vi "FGV_REWORK_records_display.vi"(7 "options":T1, 8 "error_in":errorcluster, 11 "input":variant) -> (0 "error_out":errorcluster, 3 "output":variant)   [LabVIEW 2019]
uses:
  FGV_REWORK_records_display.ctl
  REWORK_references.ctl
  REWORK_all_info.ctl
  MAIN/REWORK_header_data_display.ctl
  REWORK_gear_statuses.ctl
  REWORK_gear_station.ctl
  _misc/AULocalize/SubVIs/Get Localized Phrase Compact Interface 0D.vi
  _misc/AULocalize/SubVIs/Get Localized Phrase Compact Interface 1D.vi
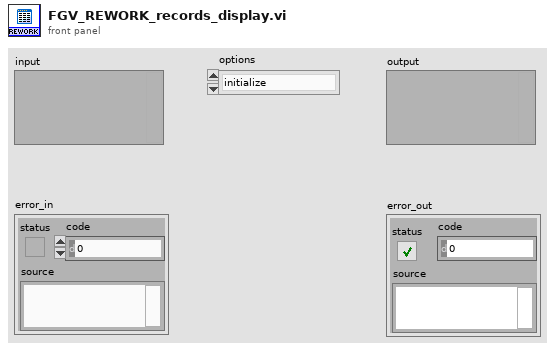
[diagram p1: front panel]
types:
  T1 = typedef "FGV_REWORK_records_display.ctl" = enum16{"initialize", "set_serial", "set_header", "set_operations", "set_results", "set_batches", "get_serial", "get_part_ID", "get_operation_IDs", "toggle_results", "show_all_results", "hide_all_results", "display", "clear"}
  T2 = typedef "REWORK_all_info.ctl" = cluster{"serial":string, "REWORK_header":T3, "operations":string[][], "operation_statuses":T4[], "results":string[][], "result_statuses":T4[], "batches":string[][], "batch_statuses":T4[], "REWORK_references":T5}
  T3 = typedef "REWORK_header_data_display.ctl" = cluster{"ID":string, "creation_time":string, "last_station":string, "last_status":string, "pinion_serial":string, "batch_code":string}
  T4 = typedef "REWORK_gear_statuses.ctl" = enum16{"OP_OK_hide", "OP_OK_show", "OP_NOK_hide", "OP_NOK_show", "OP_interrupted_hide", "OP_interrupted_show", "OP_in_operation_hide", "OP_in_operation_show", "OP_unexpected_hide", "OP_unexpected_show", "RE_REAL_OK", "RE_REAL_NOK", "RE_STRING", "RE_sub_header", "RE_no_data", "RE_unexpected", "BA_sub_header", "BA_data", "BA_no_data"}
  T5 = typedef "REWORK_references.ctl" = cluster{"front_panel_reference":refnum<vi>, "SQL_listbox_reference":refnum<vi>, "REWORK_header_data_display":refnum<vi>}
  T6 = typedef "REWORK_gear_station.ctl" = u16
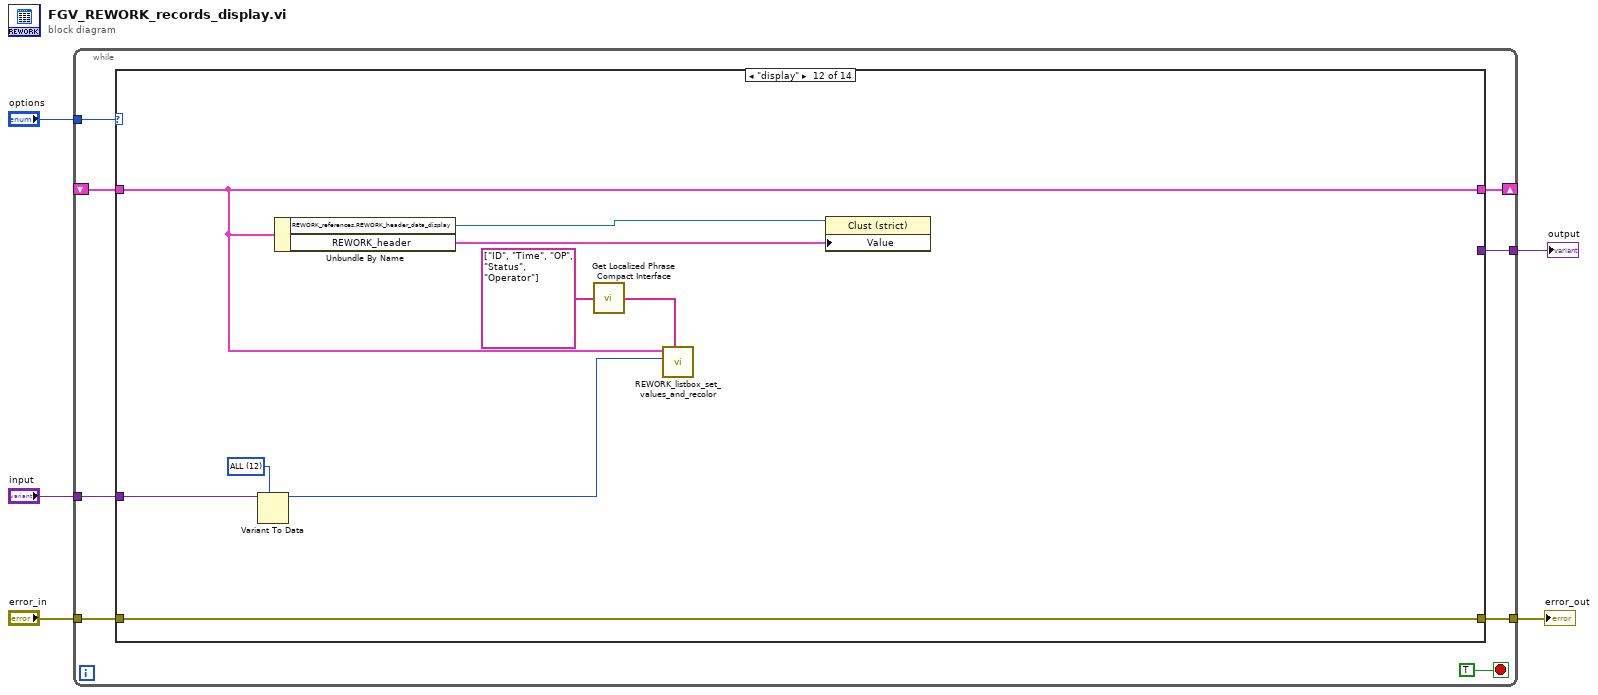
[diagram p0: block diagram]
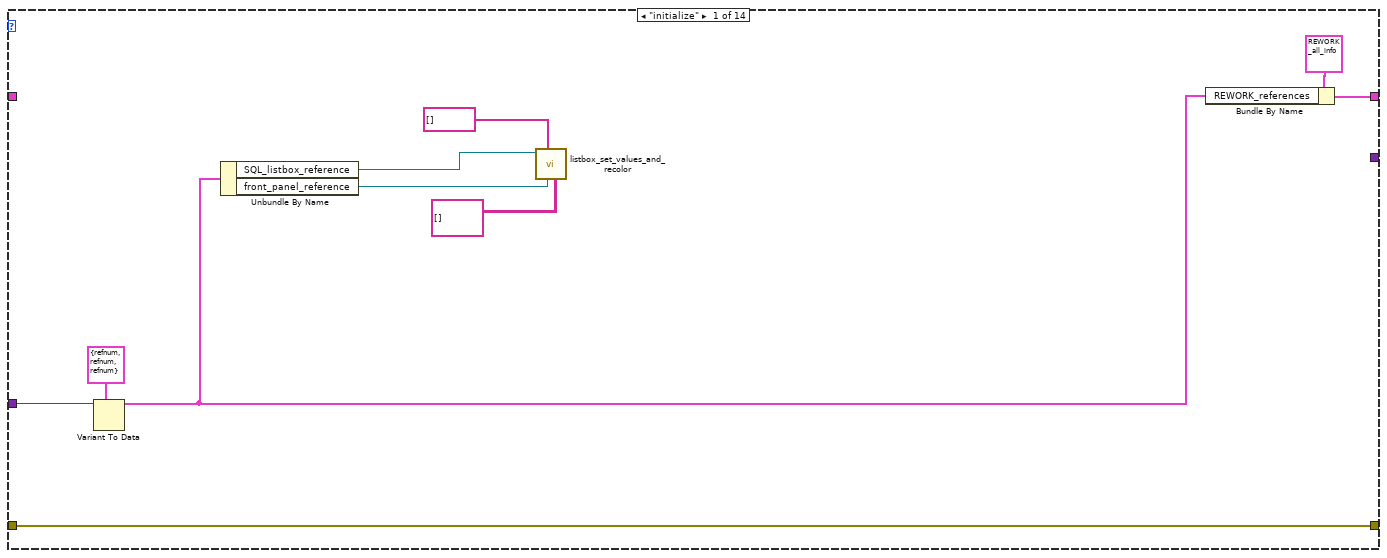
[diagram p2: hidden frame]
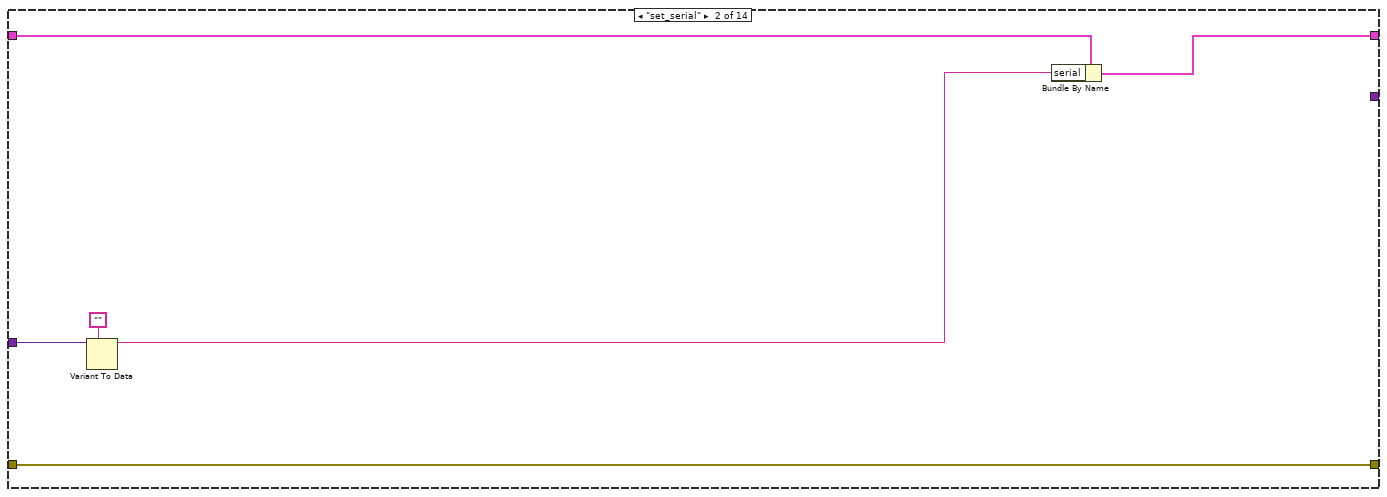
[diagram p3: hidden frame]
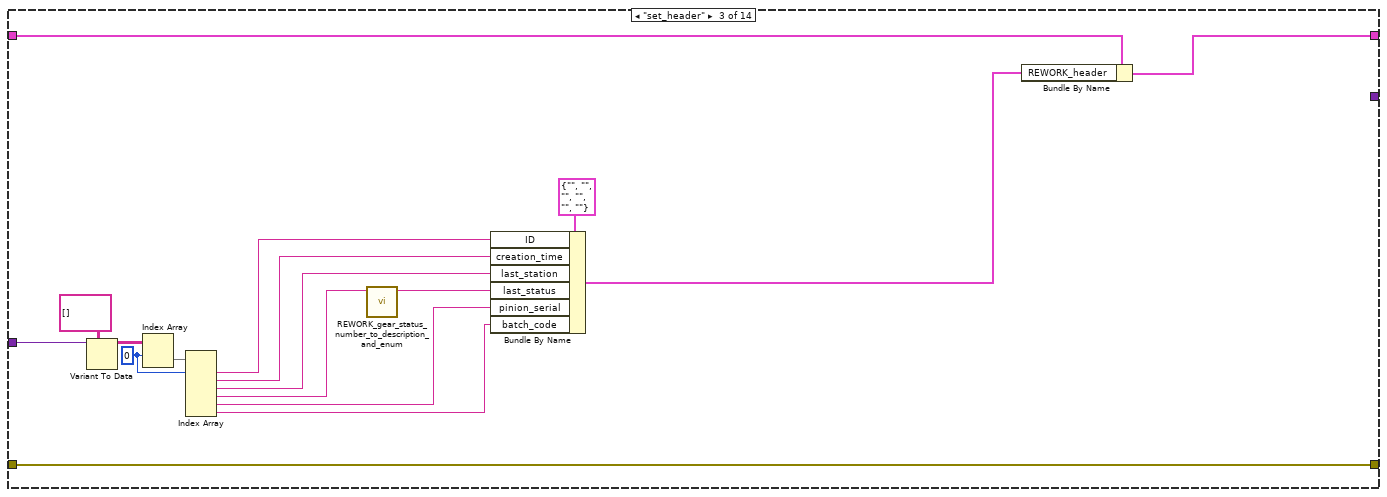
[diagram p4: hidden frame]
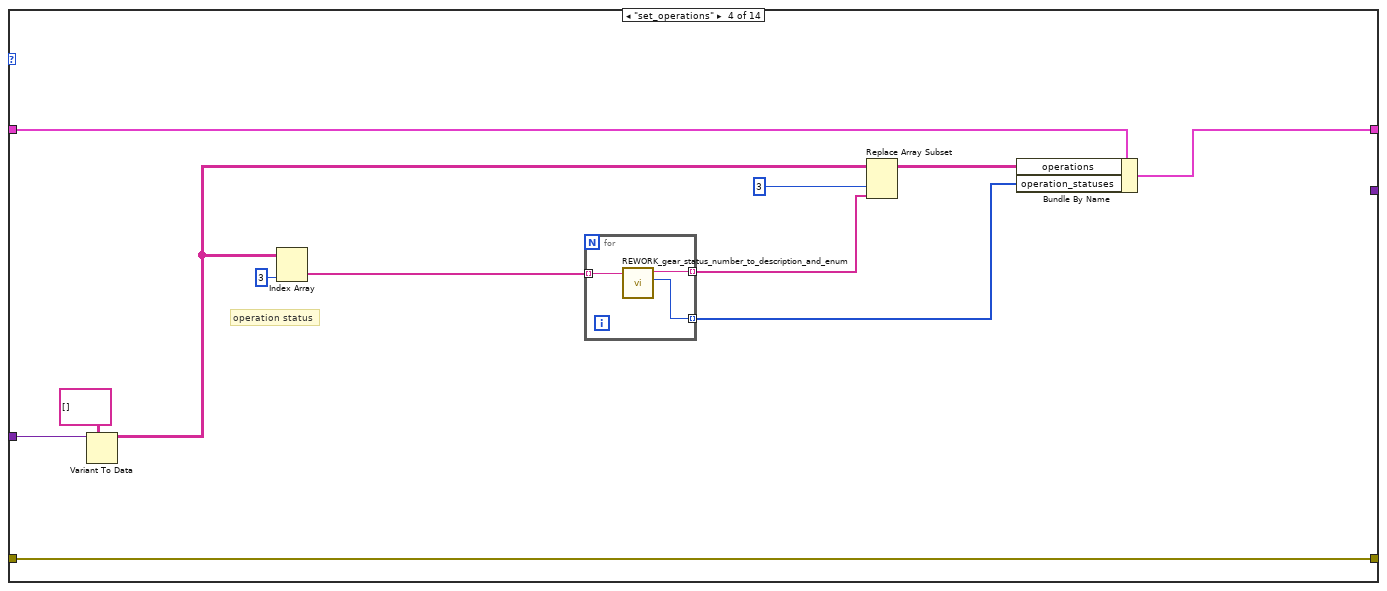
[diagram p5: hidden frame]
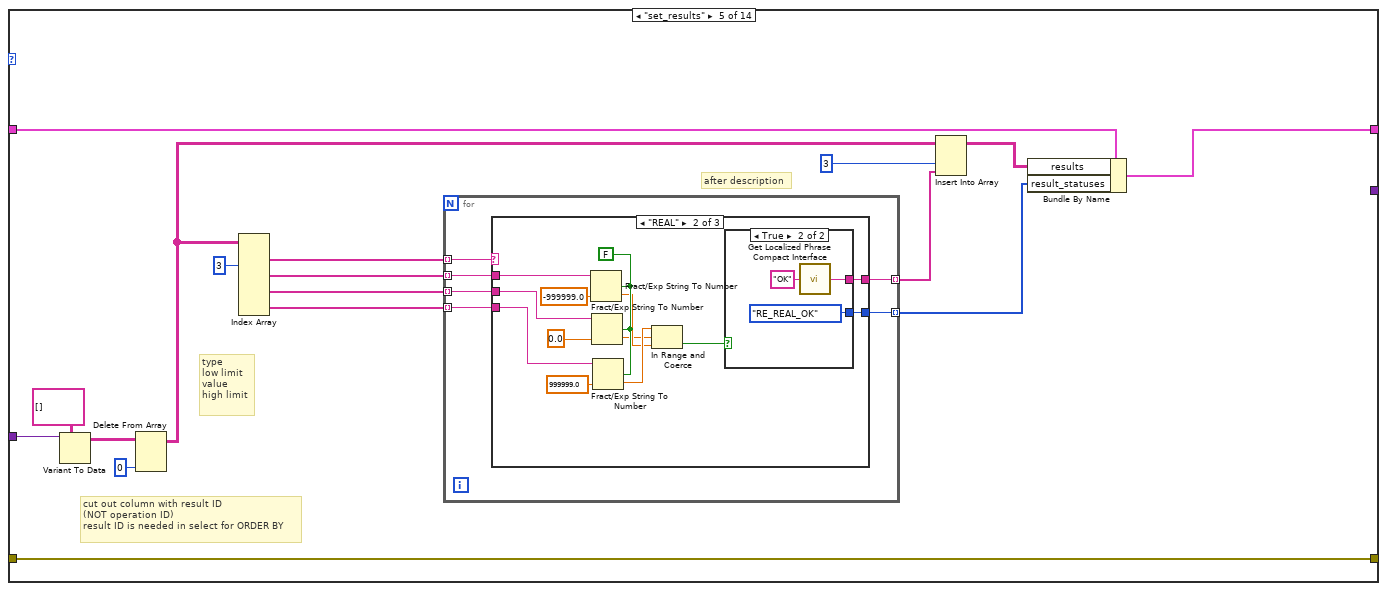
[diagram p6: hidden frame]
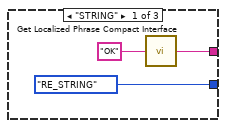
[diagram p7: hidden frame]
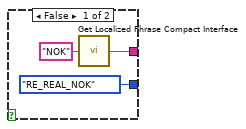
[diagram p8: hidden frame]
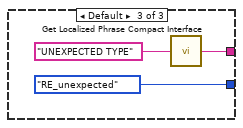
[diagram p9: hidden frame]
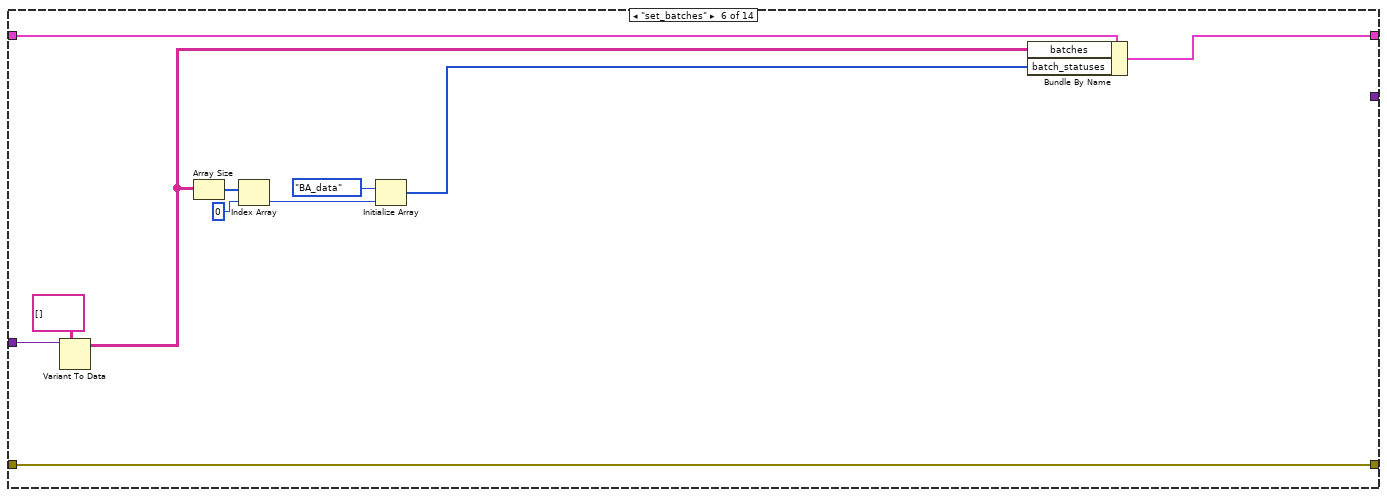
[diagram p10: hidden frame]
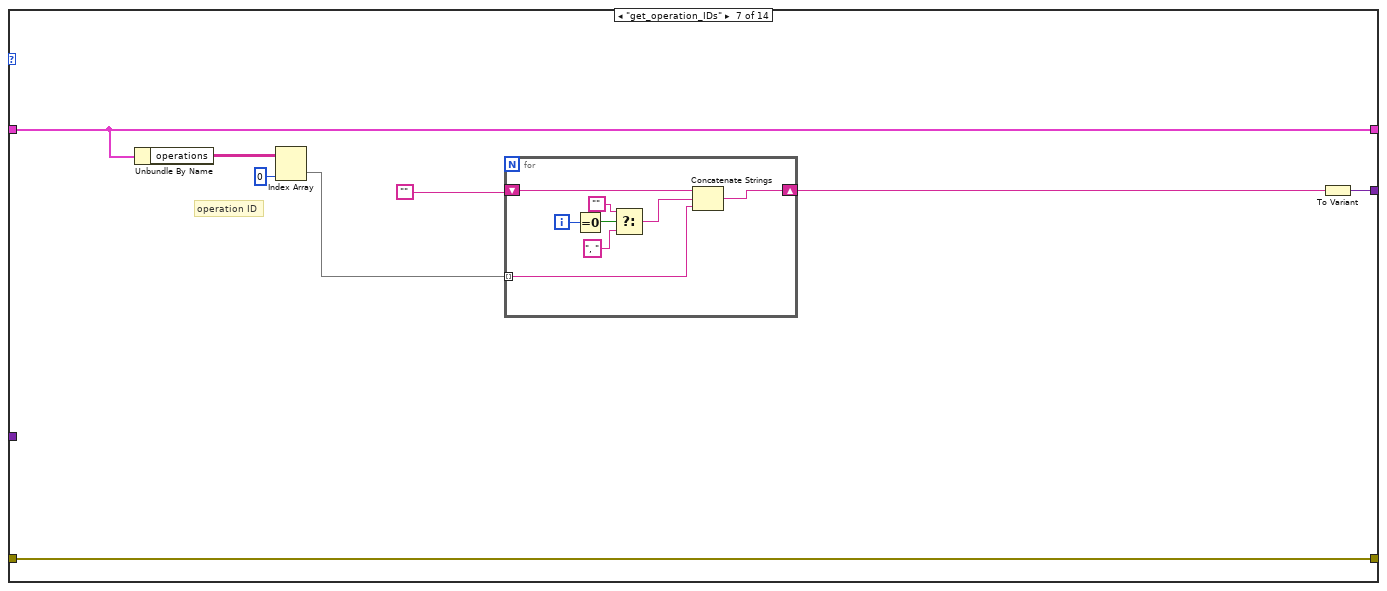
[diagram p11: hidden frame]
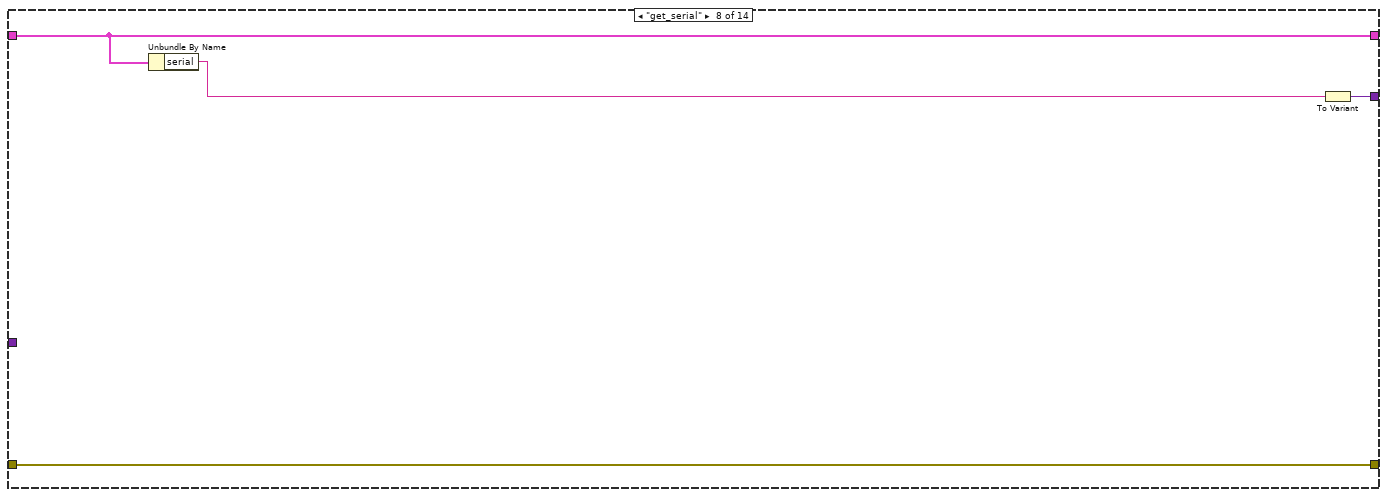
[diagram p12: hidden frame]
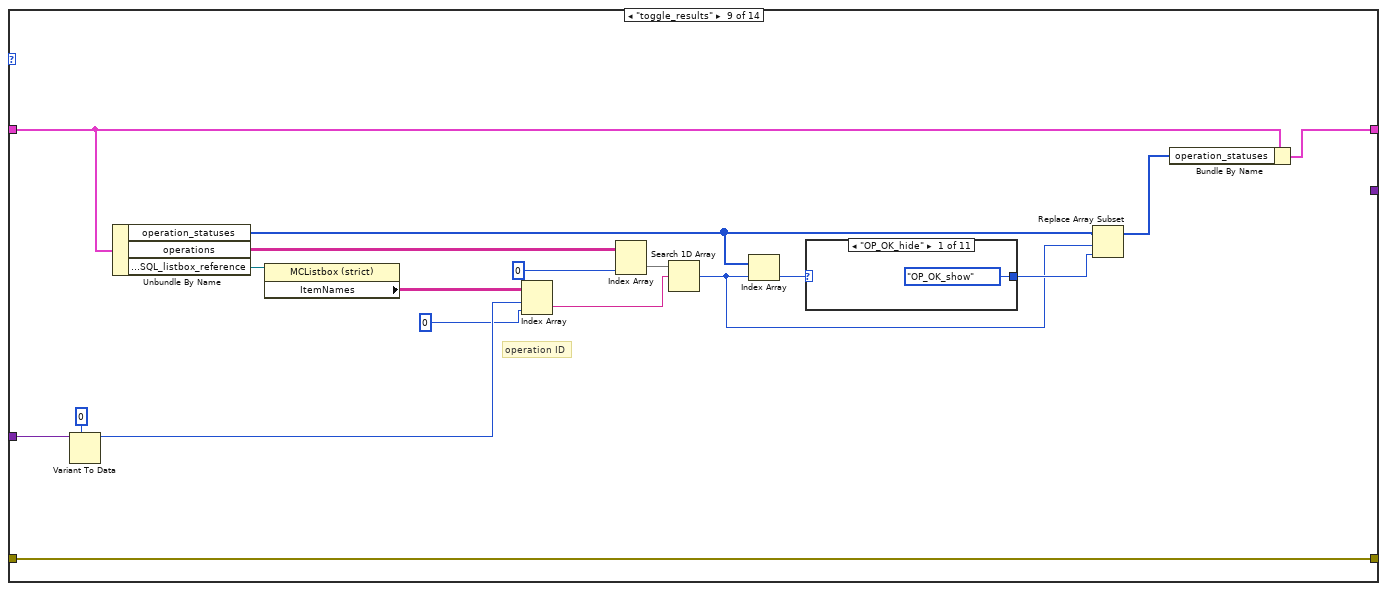
[diagram p13: hidden frame]
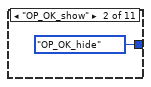
[diagram p14: hidden frame]
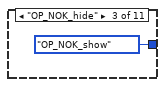
[diagram p15: hidden frame]
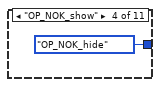
[diagram p16: hidden frame]
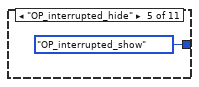
[diagram p17: hidden frame]
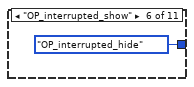
[diagram p18: hidden frame]
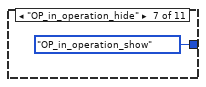
[diagram p19: hidden frame]
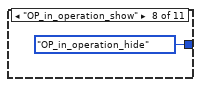
[diagram p20: hidden frame]
diagram:
  n1 = while {
    tunnel: "options" -> [w12]
    tunnel: [w11] -> w5
    tunnel: "error_in" -> [w10]
    shift-right: [w9] -> _
    shift-left: _ -> [w8]
    tunnel: "input" -> [w7]
    tunnel: [w6] -> w1
    stop <- TRUE stop-if-true
    n2 = case shown="\"display\"" w12 {
      tunnel: [w23 w29 w46 w58 w78 w120 w128 w140 w158 w174 w187 w204 w215 w216] -> w11
      tunnel: w10 -> [w23 w29 w46 w58 w78 w120 w128 w140 w158 w174 w187 w204 w215 w216]
      tunnel: [w15 w28 w45 w57 w77 w119 w126 w138 w142 w172 w185 w200 w208 w219] -> w9
      tunnel: w8 -> [_ w26 w43 w55 w75 w117 w126 w138 w143 w173 w186 w200 w212 w219]
      tunnel: w7 -> [w19 w27 w44 w56 w76 w118 _ _ w156 _ _ w199 _ _]
      tunnel: [_ _ _ _ _ _ w127 w139 _ _ _ _ _ w218] -> w6
      frame "initialize" {
        n3 = Variant To Data(type=T5 {"front_panel_reference"=refnum, "SQL_listbox_reference"=refnum, "REWORK_header_data_display"=refnum} ("REWORK_references"), Variant=w19) -> (data=w16:T5)  [unwired: 1 in, 1 out]
        n4 = Unbundle By Name(w16) -> ("SQL_listbox_reference"=w17:refnum<vi>, "front_panel_reference"=w18:refnum<vi>)
        n5 = call "listbox_set_values_and_recolor.vi"("item_names"=string[][] [], "front_panel_reference"=w18, "column_names"=string[] [], "multicolumn_listbox_reference_in"=w17) -> ()  [unwired: 6 in, 2 out]
        n6 = Bundle By Name(cluster=T2 {"serial"="", "REWORK_header"={"ID"="", "creation_time"="", "last_station"="", "last_status"="", "pinion_serial"="", "batch_code"=""}, "operations"=[], "operation_statuses"=[], "results"=[], "result_statuses"=[], "batches"=[], "batch_statuses"=[], "REWORK_references"={"front_panel_reference"=refnum, "SQL_listbox_reference"=refnum, "REWORK_header_data_display"=refnum}} ("REPORT_all_info"), "REWORK_references"=w16) -> (w15:T2)
      }
      frame "set_serial" {
        n7 = Variant To Data(type="", Variant=w27) -> (data=w24:string)  [unwired: 1 in, 1 out]
        n8 = Bundle By Name(cluster=w26, "serial"=w24) -> (w28:T2)
      }
      frame "set_header" {
        w38 = 0 ("index (row)")
        n9 = Variant To Data(type=string[][] [], Variant=w44) -> (data=w40:string[][])  [unwired: 1 in, 1 out]
        n10 = Index Array(array=w40, index (row)=w38) -> (element=w39:string[])  [unwired: 1 in]
        n11 = Index Array(array=w39, index #1=w38) -> (element #1=w36:string, element #2=w37:string, element #3=w35:string, element #4=w33:string, element #5=w34:string, element #6=w30:string)  [unwired: 5 in]
        n12 = call "REWORK_gear_status_number_to_description_and_enum.vi"("status_nmb"=w33) -> ("status_description"=w32:string)  [unwired: 9 in, 1 out]
        n13 = Bundle By Name(cluster=T3 {"ID"="", "creation_time"="", "last_station"="", "last_status"="", "pinion_serial"="", "batch_code"=""} ("REPORT_GEAR_header"), "ID"=w36, "creation_time"=w37, "last_station"=w35, "last_status"=w32, "pinion_serial"=w34, "batch_code"=w30) -> (w41:T3)
        n14 = Bundle By Name(cluster=w43, "REWORK_header"=w41) -> (w45:T2)
      }
      frame "set_operations" {
        # "operation status"
        n15 = Variant To Data(type=string[][] [], Variant=w56) -> (data=w50:string[][])  [unwired: 1 in, 1 out]
        n16 = Index Array(array=w50, index (col)=3 ("disabled index (col)")) -> (element=w52:string[])  [unwired: 1 in]
        n17 = for {
          tunnel: w52 -> [w61] mode=indexing
          tunnel: [w60] -> w51 mode=indexing
          tunnel: [w59] -> w47 mode=indexing
          n18 = call "REWORK_gear_status_number_to_description_and_enum.vi"("status_nmb"=w61) -> ("status_enum"=w60:T4, "status_description"=w59:string)  [unwired: 9 in]
        }
        n19 = Replace Array Subset(array=w50, new element=w47, index (col)=3 ("disabled index (col)")) -> (w48:string[][])  [unwired: 1 in]
        n20 = Bundle By Name(cluster=w55, "operations"=w48, "operation_statuses"=w51) -> (w57:T2)
      }
      frame "set_results" {
        # "after description"
        # "cut out column with result ID\n(NOT operation ID)\nresult ID is needed in select for ORDER BY"
        # "type\nlow limit\nvalue\nhigh limit"
        n21 = Variant To Data(type=string[][] [], Variant=w76) -> (data=w65:string[][])  [unwired: 1 in, 1 out]
        n22 = Delete From Array(array=w65, index (col)=0 ("disabled index (col)")) -> (array with subset deleted=w64:string[][])  [unwired: 2 in, 1 out]
        n23 = Index Array(array=w64, index (col) #1=3 ("disabled index (col)")) -> (element #1=w68:string[], element #2=w73:string[], element #3=w71:string[], element #4=w70:string[])  [unwired: 7 in]
        n24 = for {
          tunnel: w73 -> [w81] mode=indexing
          tunnel: [w84] -> w72 mode=indexing
          tunnel: [w83] -> w66 mode=indexing
          tunnel: w71 -> [w80] mode=indexing
          tunnel: w70 -> [w79] mode=indexing
          tunnel: w68 -> [w82] mode=indexing
          n25 = case shown="\"REAL\"" w82 {
            tunnel: [REWORK_gear_statuses."RE_STRING" ("REPORT_GEAR_statuses") w100 REWORK_gear_statuses."RE_unexpected" ("REPORT_GEAR_statuses")] -> w84
            tunnel: [w85 w99 w107] -> w83
            tunnel: w81 -> [_ w98 _]
            tunnel: w80 -> [_ w96 _]
            tunnel: w79 -> [_ w95 _]
            frame "STRING" {
              n26 = call-poly "Get Localized Phrase Compact Interface.vi"("Key"="OK") -> ("Translated Phrase"=w85:string)
            }
            frame "REAL" {
              w97 = FALSE ("use system decimal point (T)")
              n27 = Fract/Exp String To Number(use system decimal point (T)=w97, string=w98, default (0 dbl)=sgl -999999.0 ("default (0 DBL)")) -> (number=w93:sgl)  [unwired: 1 in, 1 out]
              n28 = Fract/Exp String To Number(use system decimal point (T)=w97, string=w96, default (0 dbl)=sgl 0.0 ("default (0 DBL)")) -> (number=w92:sgl)  [unwired: 1 in, 1 out]
              n29 = Fract/Exp String To Number(use system decimal point (T)=w97, string=w95, default (0 dbl)=sgl 999999.0 ("default (0 DBL)")) -> (number=w94:sgl)  [unwired: 1 in, 1 out]
              n30 = In Range and Coerce(upper limit=w94, x=w92, lower limit=w93) -> (In Range?=w91:bool)  [unwired: 1 out]
              n31 = case shown="True" w91 {
                tunnel: [REWORK_gear_statuses."RE_REAL_NOK" ("REPORT_GEAR_statuses") REWORK_gear_statuses."RE_REAL_OK" ("REPORT_GEAR_statuses")] -> w100
                tunnel: [w101 w104] -> w99
                frame False {
                  n32 = call-poly "Get Localized Phrase Compact Interface.vi"("Key"="NOK") -> ("Translated Phrase"=w101:string)
                }
                frame True {
                  n33 = call-poly "Get Localized Phrase Compact Interface.vi"("Key"="OK") -> ("Translated Phrase"=w104:string)
                }
              }
            }
            frame Default {
              n34 = call-poly "Get Localized Phrase Compact Interface.vi"("Key"="UNEXPECTED TYPE") -> ("Translated Phrase"=w107:string)
            }
          }
        }
        n35 = Insert Into Array(array=w64, index (col)=3 ("disabled index (col)"), new element=w66) -> (w67:string[][])  [unwired: 1 in]
        n36 = Bundle By Name(cluster=w75, "results"=w67, "result_statuses"=w72) -> (w77:T2)
      }
      frame "set_batches" {
        n37 = Variant To Data(type=string[][] [], Variant=w118) -> (data=w114:string[][])  [unwired: 1 in, 1 out]
        n38 = Array Size(array=w114) -> (size(s)=w113:i32[])
        n39 = Index Array(array=w113, index=0) -> (element=w111:i32)
        n40 = Initialize Array(REWORK_gear_statuses."BA_data" ("REPORT_GEAR_statuses"), w111) -> (w110:T4[])
        n41 = Bundle By Name(cluster=w117, "batches"=w114, "batch_statuses"=w110) -> (w119:T2)
      }
      frame "get_operation_IDs" {
        # "operation ID"
        n42 = Unbundle By Name(w126) -> ("operations"=w125:string[][])
        n43 = Index Array(array=w125, index (col)=0 ("disabled index (col)")) -> (element=w123:string[])  [unwired: 1 in]
        n44 = for {
          tunnel: w123 -> [w129] mode=indexing
          shift-right: [w132] -> w121
          shift-left: "" -> [w131]
          i -> [w133]
          n45 = Equal To 0?(x=w133) -> (x = 0?=w134:bool)
          n46 = Select(t="", s=w134, f=", ") -> (s? t:f=w130:string)
          n47 = Concatenate Strings(w131, w130, w129) -> (w132:string)
        }
        n48 = To Variant(anything=w121) -> (Variant=w127:variant)
      }
      frame "get_serial" {
        n49 = Unbundle By Name(w138) -> ("serial"=w137:string)
        n50 = To Variant(anything=w137) -> (Variant=w139:variant)
      }
      frame "toggle_results" {
        # "operation ID"
        n51 = Variant To Data(type=0 ("Row"), Variant=w156) -> (data=w153:i32)  [unwired: 1 in, 1 out]
        n52 = Unbundle By Name(w143) -> ("operation_statuses"=w146:T4[], "operations"=w151:string[][], "REWORK_references.SQL_listbox_reference"=w157:refnum<vi>)
        n53 = property class="MCListbox (strict)"(reference=w157) -> ("ItemNames"=w154:string[][])  [unwired: 1 in, 2 out]
        n54 = Index Array(array=w154, index (row)=w153, index (col)=0 ("disabled index (col)")) -> (element=w148:string)
        n55 = Index Array(array=w151, index (col)=0 ("disabled index (col)")) -> (element=w149:string[])  [unwired: 1 in]
        n56 = Search 1D Array(1D array=w149, element=w148) -> (index of element=w144:i32)  [unwired: 1 in]
        n57 = Index Array(array=w146, index=w144) -> (element=w147:T4)
        n58 = case shown="\"OP_OK_hide\"" w147 {
          selector: w147 -> [_ _ _ _ _ _ _ _ _ _ w169]
          tunnel: [REWORK_gear_statuses."OP_OK_show" ("REPORT_GEAR_statuses") REWORK_gear_statuses."OP_OK_hide" ("REPORT_GEAR_statuses") REWORK_gear_statuses."OP_NOK_show" ("REPORT_GEAR_statuses") REWORK_gear_statuses."OP_NOK_hide" ("REPORT_GEAR_statuses") REWORK_gear_statuses."OP_interrupted_show" ("REPORT_GEAR_statuses") REWORK_gear_statuses."OP_interrupted_hide" ("REPORT_GEAR_statuses") REWORK_gear_statuses."OP_in_operation_show" ("REPORT_GEAR_statuses") REWORK_gear_statuses."OP_in_operation_hide" ("REPORT_GEAR_statuses") REWORK_gear_statuses."OP_unexpected_show" ("REPORT_GEAR_statuses") REWORK_gear_statuses."OP_unexpected_hide" ("REPORT_GEAR_statuses") w169] -> w145
          frame "OP_OK_hide" {
          }
          frame "OP_OK_show" {
          }
          frame "OP_NOK_hide" {
          }
          frame "OP_NOK_show" {
          }
          frame "OP_interrupted_hide" {
          }
          frame "OP_interrupted_show" {
          }
          frame "OP_in_operation_hide" {
          }
          frame "OP_in_operation_show" {
          }
          frame "OP_unexpected_hide" {
          }
          frame "OP_unexpected_show" {
          }
          frame Default {
          }
        }
        n59 = Replace Array Subset(array=w146, new element=w145, index=w144) -> (w141:T4[])
        n60 = Bundle By Name(cluster=w143, "operation_statuses"=w141) -> (w142:T2)
      }
      frame "show_all_results" {
        n61 = Unbundle By Name(w173) -> ("operation_statuses"=w171:T4[])
        n62 = for {
          tunnel: w171 -> [w176] mode=indexing
          tunnel: [w175] -> w170 mode=indexing
          n63 = case shown="Default" w176 {
            selector: w176 -> [_ _ _ _ _ w182]
            tunnel: [REWORK_gear_statuses."OP_OK_show" ("REPORT_GEAR_statuses") REWORK_gear_statuses."OP_NOK_show" ("REPORT_GEAR_statuses") REWORK_gear_statuses."OP_interrupted_show" ("REPORT_GEAR_statuses") REWORK_gear_statuses."OP_in_operation_show" ("REPORT_GEAR_statuses") REWORK_gear_statuses."OP_unexpected_show" ("REPORT_GEAR_statuses") w182] -> w175
            frame "OP_OK_hide" {
            }
            frame "OP_NOK_hide" {
            }
            frame "OP_interrupted_hide" {
            }
            frame "OP_in_operation_hide" {
            }
            frame "OP_unexpected_hide" {
            }
            frame Default {
            }
          }
        }
        n64 = Bundle By Name(cluster=w173, "operation_statuses"=w170) -> (w172:T2)
      }
      frame "hide_all_results" {
        n65 = Unbundle By Name(w186) -> ("operation_statuses"=w184:T4[])
        n66 = for {
          tunnel: w184 -> [w188] mode=indexing
          tunnel: [w189] -> w183 mode=indexing
          n67 = case shown="\"OP_unexpected_show\"" w188 {
            selector: w188 -> [_ _ _ _ _ w195]
            tunnel: [REWORK_gear_statuses."OP_OK_hide" ("REPORT_GEAR_statuses") REWORK_gear_statuses."OP_NOK_hide" ("REPORT_GEAR_statuses") REWORK_gear_statuses."OP_interrupted_hide" ("REPORT_GEAR_statuses") REWORK_gear_statuses."OP_in_operation_hide" ("REPORT_GEAR_statuses") REWORK_gear_statuses."OP_unexpected_hide" ("REPORT_GEAR_statuses") w195] -> w189
            frame "OP_OK_show" {
            }
            frame "OP_NOK_show" {
            }
            frame "OP_interrupted_show" {
            }
            frame "OP_in_operation_show" {
            }
            frame "OP_unexpected_show" {
            }
            frame Default {
            }
          }
        }
        n68 = Bundle By Name(cluster=w186, "operation_statuses"=w183) -> (w185:T2)
      }
      frame "display" {
        w197 = T6 12 items=["Station 10", "Station 20", "Station 30", "Station 40", "Station 50", "Station 60", "Station 70", "Station 80", "Station 90", "Station 100", "Station 110", "Station 120", "ALL"] ("REPORT_GEAR_station")
        n69 = Variant To Data(type=w197, Variant=w199) -> (data=w198:T6)  [unwired: 1 in, 1 out]
        n70 = Unbundle By Name(w200) -> ("REWORK_references.REWORK_header_data_display"=w203:refnum<vi>, "REWORK_header"=w202:T3)
        n71 = call-poly "Get Localized Phrase Compact Interface.vi"("Key"=string[] ["ID", "Time", "OP", "Status", "Operator"] ("column_names")) -> ("Translated Phrase"=w196:string[])
        n72 = call "REWORK_listbox_set_values_and_recolor.vi"("column_names"=w196, "REPORT_GEAR_station"=w198, "REPORT_all_info"=w200) -> ()  [unwired: 8 in, 1 out]
        n73 = property class="Clust (strict)"(reference=w203, "Value"=w202) -> ()  [unwired: 1 in, 2 out]
      }
      frame "clear" {
        n74 = Unbundle By Name(w212) -> ("REWORK_references"=w209:T5, "REWORK_references.SQL_listbox_reference"=w211:refnum<vi>, "REWORK_references.front_panel_reference"=w210:refnum<vi>, "REWORK_references.REWORK_header_data_display"=w206:refnum<vi>)
        n75 = property class="Clust (strict)"(reference=w206, "Value"=T3 {"ID"="", "creation_time"="", "last_station"="", "last_status"="", "pinion_serial"="", "batch_code"=""} ("REPORT_GEAR_header")) -> ()  [unwired: 1 in, 2 out]
        n76 = call "listbox_set_values_and_recolor.vi"("item_names"=string[][] [], "front_panel_reference"=w210, "column_names"=string[] [], "multicolumn_listbox_reference_in"=w211) -> ()  [unwired: 6 in, 2 out]
        n77 = Bundle By Name(cluster=T2 {"serial"="", "REWORK_header"={"ID"="", "creation_time"="", "last_station"="", "last_status"="", "pinion_serial"="", "batch_code"=""}, "operations"=[], "operation_statuses"=[], "results"=[], "result_statuses"=[], "batches"=[], "batch_statuses"=[], "REWORK_references"={"front_panel_reference"=refnum, "SQL_listbox_reference"=refnum, "REWORK_header_data_display"=refnum}} ("REPORT_all_info"), "REWORK_references"=w209) -> (w208:T2)
      }
      frame "get_part_ID" {
        n78 = Unbundle By Name(w219) -> ("REWORK_header.ID"=w217:string)
        n79 = To Variant(anything=w217) -> (Variant=w218:variant)
      }
    }
  }
  "error_out" <- w5
  "output" <- w1
